vi "Global_Valves.vi"() -> ()   [LabVIEW 2016]
panel:
  out "Global valve 16":bool
  out "Global valve 15":bool
  out "Global valve 14":bool
  out "Global valve 13":bool
  out "Global valve 12":bool
  out "Global valve 11":bool
  out "Global valve 10":bool
  out "Global valve 9":bool
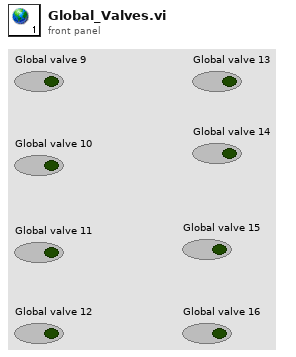
[diagram p1: front panel]
diagram:
